vi "Calculate_Obstace_Coordinates.vi"(8 "error in (no error)":errorcluster, 9 "angles[]":dbl[](array[numeric]), 10 "distance[]":dbl[](array[numeric]), 11 "Current_Position":T1) -> (0 "error out":errorcluster, 1 "Y Out":dbl[](array[numeric]), 2 "X Out":dbl[](array[numeric]), 4 "detected?":bool[](array[boolean]))   [LabVIEW 2017]
doc: "Calculate Obstacle coordinates from obstacles distances and angles and current robot position\ndetected? is TRUE when obstacle distance is within sensor range, FALSE when it is NaN or out of range"
uses:
  Ctl/Current_Position.ctl
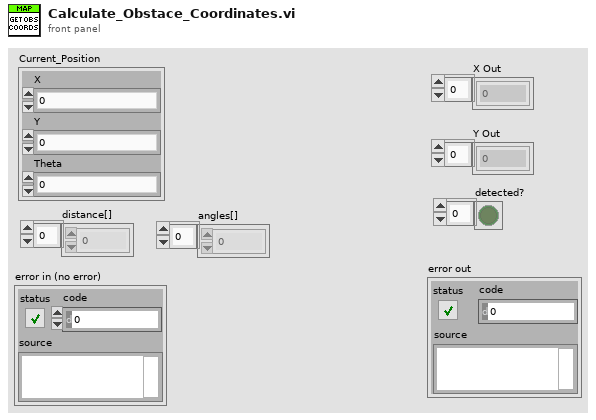
[diagram p1: front panel]
types:
  T1 = typedef "Current_Position.ctl" = cluster{"X":dbl, "Y":dbl, "Theta":dbl}
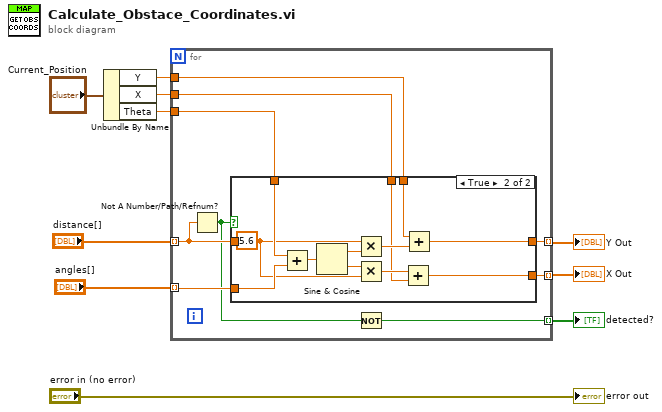
[diagram p0: block diagram]
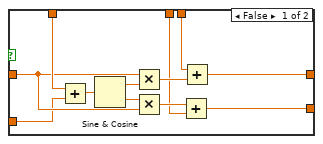
[diagram p2: hidden frame]
diagram:
  n1 = Unbundle By Name("Current_Position") -> ("Y"=w7:dbl, "X"=w6:dbl, "Theta"=w5:dbl)
  n2 = for {
    tunnel: w7 -> [w16]
    tunnel: w6 -> [w17]
    tunnel: w5 -> [w15]
    tunnel: [w19] -> w2 mode=indexing
    tunnel: [w18] -> w9 mode=indexing
    tunnel: "distance[]" -> [w13] mode=indexing
    tunnel: "angles[]" -> [w14] mode=indexing
    tunnel: [w11] -> w1 mode=indexing
    n3 = Not A Number/Path/Refnum?(number/path/refnum=w13) -> (NaN/Path/Refnum?=w12:bool)
    n4 = case shown="True" w12 {
      tunnel: [w26 w38] -> w19
      tunnel: [w25 w37] -> w18
      tunnel: w17 -> [w24 w36]
      tunnel: w16 -> [w23 w35]
      tunnel: w15 -> [w22 w34]
      tunnel: w13 -> [w21 _]
      tunnel: w14 -> [w20 w33]
      frame False {
        n5 = Add(x=w22, y=w20) -> (x+y=w31:dbl)
        n6 = Sine & Cosine(0:w31) -> (1:w30:dbl, 2:w29:dbl)
        n7 = Multiply(x=w21, y=w30) -> (x*y=w28:dbl)
        n8 = Multiply(x=w29, y=w21) -> (x*y=w27:dbl)
        n9 = Add(x=w27, y=w24) -> (x+y=w25:dbl)
        n10 = Add(x=w23, y=w28) -> (x+y=w26:dbl)
      }
      frame True {
        w32 = 5.6 ("x")
        n11 = Add(x=w34, y=w33) -> (x+y=w43:dbl)
        n12 = Sine & Cosine(0:w43) -> (1:w42:dbl, 2:w41:dbl)
        n13 = Multiply(x=w32, y=w42) -> (x*y=w40:dbl)
        n14 = Multiply(x=w41, y=w32) -> (x*y=w39:dbl)
        n15 = Add(x=w39, y=w36) -> (x+y=w37:dbl)
        n16 = Add(x=w35, y=w40) -> (x+y=w38:dbl)
      }
    }
    n17 = Not(x=w12) -> (.not. x?=w11:bool)
  }
  "Y Out" <- w2
  "X Out" <- w9
  "detected?" <- w1
  "error out" <- "error in (no error)"
